vi "题目 4.vi"() -> ()   [LabVIEW 2017]
uses:
  <vilib>/Analysis/2dsp.llb/Real FFT.vi
  <vilib>/measure/NI_MABase.lvlib
  <vilib>/Analysis/NI_AALPro.lvlib
panel:
  in  "sampling info":cluster{"Fs":dbl, "#s":dbl}={"Fs"=1000.0, "#s"=1000.0} caption="采样信息" {"Fs" format="%.2p"}
  out "时域信号":dbl[](graph)
  out "频域信号":dbl[](graph)
  in  "amplitude3":dbl=1.0 caption="幅值3" format="%0.2p"
  in  "frequency3":dbl=10.0 caption="频率3" format="%0.2p"
  in  "amplitude2":dbl=1.0 caption="幅值2" format="%0.2p"
  in  "frequency2":dbl=10.0 caption="频率2" format="%0.2p"
  in  "amplitude1":dbl=1.0 caption="幅值1" format="%0.2p"
  in  "frequency1":dbl=10.0 caption="频率1" format="%0.2p"
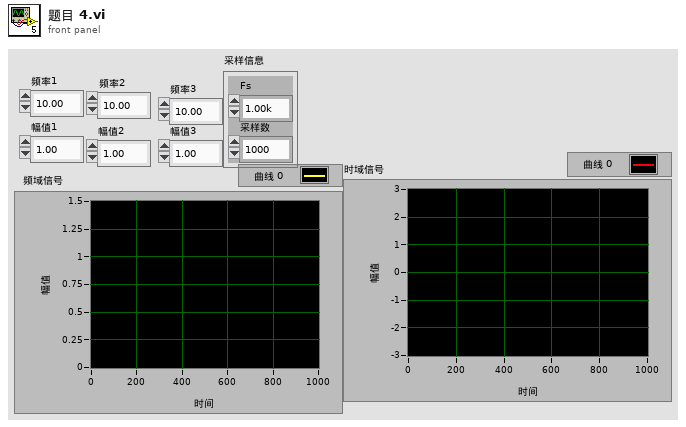
[diagram p1: front panel]
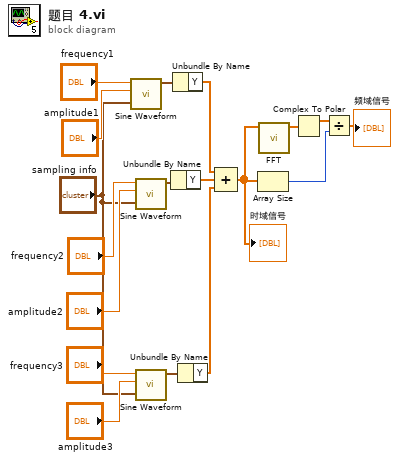
[diagram p0: block diagram]
diagram:
  n1 = call <vilib>:"Sine Waveform.vi"("sampling info"="sampling info", "amplitude"="amplitude1", "frequency"="frequency1") -> ("signal out"=w12:waveform(dbl))  [unwired: 7 in, 1 out]
  n2 = call <vilib>:"Sine Waveform.vi"("sampling info"="sampling info", "amplitude"="amplitude2", "frequency"="frequency2") -> ("signal out"=w11:waveform(dbl))  [unwired: 7 in, 1 out]
  n3 = call <vilib>:"Sine Waveform.vi"("sampling info"="sampling info", "amplitude"="amplitude3", "frequency"="frequency3") -> ("signal out"=w10:waveform(dbl))  [unwired: 7 in, 1 out]
  n4 = Unbundle By Name(w11) -> ("Y"=w8:dbl[])
  n5 = Unbundle By Name(w12) -> ("Y"=w9:dbl[])
  n6 = Unbundle By Name(w10) -> ("Y"=w7:dbl[])
  n7 = Compound Arithmetic op=ADD(w9, w8, w7) -> (w4:dbl[])
  "时域信号" <- w4
  n8 = Array Size(array=w4) -> (size(s)=w1:i32)
  n9 = call-poly <vilib>:"FFT.vi"("X"=w4) -> ("FFT {X}"=w3:cdb[])  [unwired: 9 in, 1 out]
  n10 = Complex To Polar(r * e^(i*theta)=w3) -> (r=w6:dbl[])  [unwired: 1 out]
  n11 = Divide(x=w6, y=w1) -> (x/y=→"频域信号":dbl[])
